vi "Update Timing Config.vi"(7 "Timing Engine":T1=enum."Low Speed", 8 "error in (no error)":errorcluster, 10 "Timing Cfg":T2, 11 "FP Controls in":refnum<class "FP Controls.lvclass">) -> (0 "error out":errorcluster, 3 "FP Controls out":refnum<class "FP Controls.lvclass">)   [LabVIEW 2012, in "Configuration Grandmaster.lvlib" / "FP Controls.lvclass"]
uses:
  FP Controls.lvclass
  Common/Controls/Group Timing Info.ctl
  Common/Controls/TE_Designator.ctl
  FP Controls.lvclass/FP Controls.ctl
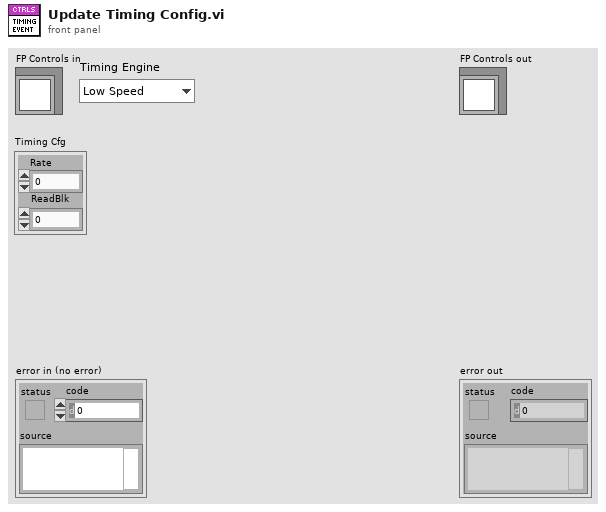
[diagram p1: front panel]
types:
  T1 = typedef "TE_Designator.ctl" = enum16{"High Speed", "Low Speed"}
  T2 = typedef "Group Timing Info.ctl" = cluster{"Rate":dbl, "ReadBlk":i32}
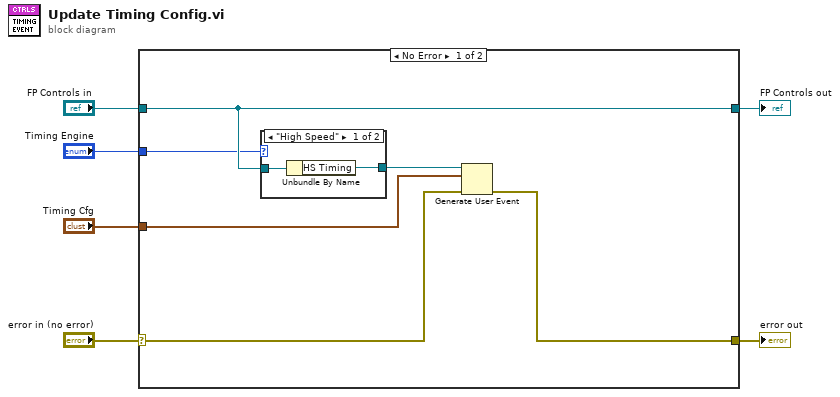
[diagram p0: block diagram]
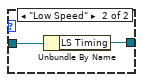
[diagram p2: hidden frame]
diagram:
  n1 = case shown="No Error" "error in (no error)" {
    selector: "error in (no error)" -> [w8 w18]
    tunnel: [w7 w18] -> w5
    tunnel: [w12 w17] -> w3
    tunnel: "FP Controls in" -> [w12 w17]
    tunnel: "Timing Engine" -> [w11 _]
    tunnel: "Timing Cfg" -> [w9 _]
    frame No Error {
      n2 = case shown="\"High Speed\"" w11 {
        tunnel: w12 -> [w14 w16]
        tunnel: [w13 w15] -> w10
        frame "High Speed" {
          n3 = Unbundle By Name(w14) -> ("HS Timing"=w13:refnum<user-event>)
        }
        frame "Low Speed" {
          n4 = Unbundle By Name(w16) -> ("LS Timing"=w15:refnum<user-event>)
        }
      }
      n5 = Generate User Event(user event=w10, event data cluster=w9, error in=w8) -> (error out=w7:errorcluster)  [unwired: 1 out]
    }
    frame Error {
    }
  }
  "error out" <- w5
  "FP Controls out" <- w3
